vi "connectionTest.vi"() -> (0 "error out":errorcluster, 3 "response":string)   [LabVIEW 2017]
uses:
  <vilib>/addons/InsightCM/MessageBus/Base/controls/ConnectionInfo.ctl
  <vilib>/httpClient/LabVIEWHTTPClient.lvlib
panel:
  in  "TransceiverPort":u16=6342
  in  "ClientName":string="Bop9068"
  in  "TrannsceiverHost":string="10.2.64.56"
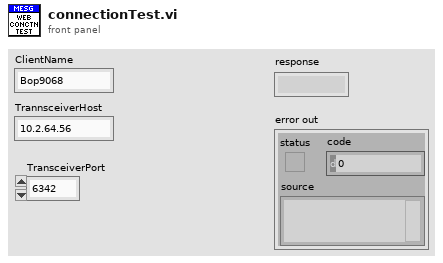
[diagram p1: front panel]
types:
  T1 = typedef "ConnectionInfo.ctl" = cluster{"ClientName":string, "TransceiverHost":string, "TransceiverPort":u16, "Password":string}
  T2 = typedef "LabVIEWHTTPClient.lvlib/ClientHandle.ctl" = refnum<k1>
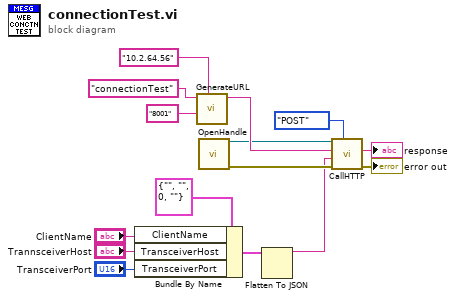
[diagram p0: block diagram]
diagram:
  n1 = Bundle By Name(cluster=T1 {"ClientName"="", "TransceiverHost"="", "TransceiverPort"=0, "Password"=""} ("ConnInfo"), "ClientName"="ClientName", "TransceiverHost"="TrannsceiverHost", "TransceiverPort"="TransceiverPort") -> (w6:T1)
  n2 = call "GenerateURL.vi"("host"="10.2.64.56", "port"="8001", "method"="connectionTest") -> ("url"=w14:string)  [unwired: 7 in, 1 out]
  n3 = call <vilib>:"OpenHandle.vi"() -> ("client handle out"=w13:T2, "error out"=w12:errorcluster)  [unwired: 14 in]
  n4 = Flatten To JSON(anything=w6) -> (JSON string=w5:string)  [unwired: 2 in, 1 out]
  n5 = call "CallHTTP.vi"("Enum"=enum16{"GET", "POST", "DELETE"}."POST", "error in (no error)"=w12, "data"=w5, "url"=w14, "client handle"=w13) -> ("error out"=→"error out":errorcluster, "response"=→"response":string)  [unwired: 3 in, 2 out]
